vi "Control.vi"(6 "Kp2":dbl, 7 "Q":dbl, 9 "KV":dbl, 10 "Zigmae":dbl[](array[numeric]), 11 "Vr/Wr":dbl[](array[numeric])) -> (2 "W":dbl, 3 "V":dbl)   [LabVIEW 2011]
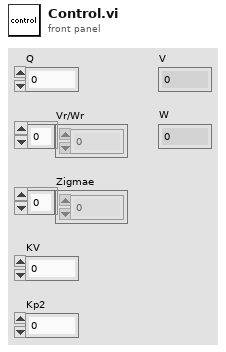
[diagram p1: front panel]
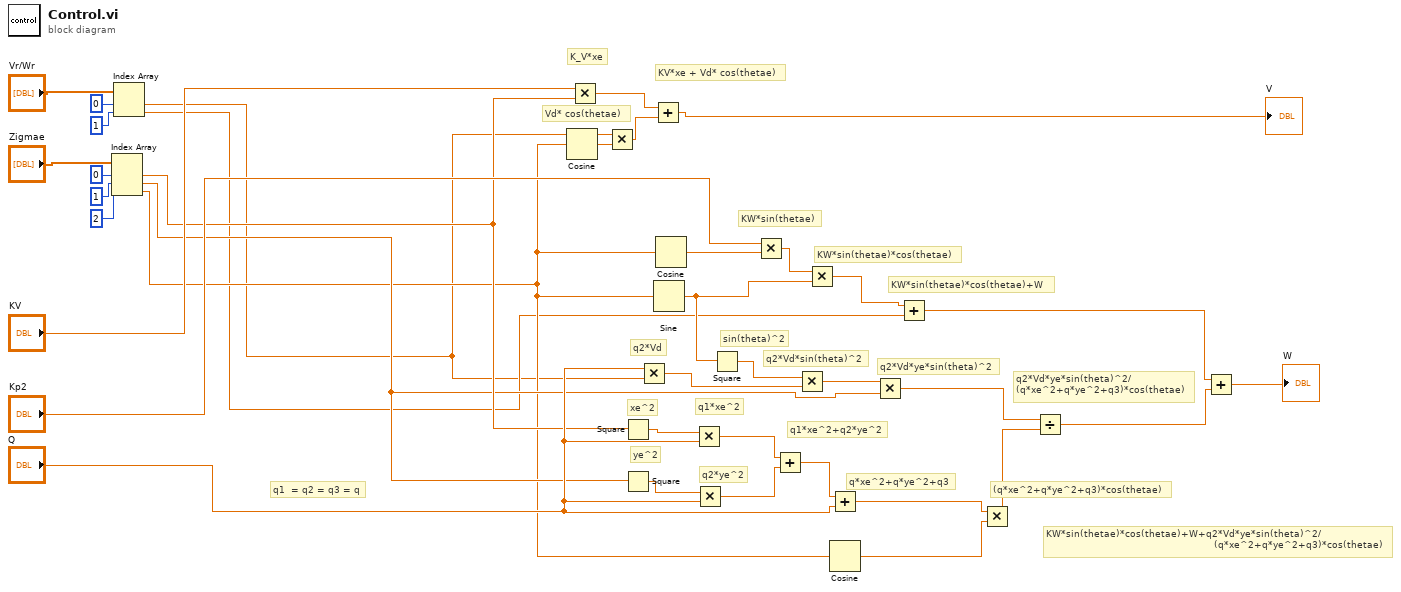
[diagram p0: block diagram]
diagram:
  # "q2*Vd*ye*sin(theta)^2"
  # "KW*sin(thetae)*cos(thetae)+W+q2*Vd*ye*sin(theta)^2/\n                                                        (q*xe^2+q*ye^2+q3)*cos(thetae)"
  # "q2*Vd*ye*sin(theta)^2/\n(q*xe^2+q*ye^2+q3)*cos(thetae)"
  # "(q*xe^2+q*ye^2+q3)*cos(thetae)"
  # "q*xe^2+q*ye^2+q3"
  # "q1*xe^2+q2*ye^2"
  # "q2*ye^2"
  # "q1*xe^2"
  # "ye^2"
  # "xe^2"
  # "q2*Vd*sin(theta)^2"
  # "sin(theta)^2"
  # "q2*Vd"
  # "q1  = q2 = q3 = q"
  # "KW*sin(thetae)*cos(thetae)+W"
  # "KW*sin(thetae)*cos(thetae)"
  # "KW*sin(thetae)"
  # "Vd* cos(thetae)"
  # "KV*xe + Vd* cos(thetae)"
  # "K_V*xe"
  n1 = Index Array(array="Zigmae", index #1=0 ("index"), index #2=1 ("index"), index #3=2 ("index")) -> (element #1=w7:dbl, element #2=w6:dbl, element #3=w5:dbl)
  n2 = Index Array(array="Vr/Wr", index #1=0 ("index"), index #2=1 ("index")) -> (element #1=w3:dbl, element #2=w4:dbl)
  n3 = Cosine(x=w5) -> (cos(x)=w14:dbl)
  n4 = Multiply(x="KV", y=w7) -> (x*y=w13:dbl)
  n5 = Multiply(x=w3, y=w14) -> (x*y=w15:dbl)
  n6 = Square(x=w7) -> (x^2=w22:dbl)
  n7 = Square(x=w6) -> (x^2=w23:dbl)
  n8 = Multiply(x="Q", y=w3) -> (x*y=w21:dbl)
  n9 = Add(x=w13, y=w15) -> (x+y=→"V":dbl)
  n10 = Sine(x=w5) -> (sin(x)=w19:dbl)
  n11 = Cosine(x=w5) -> (cos(x)=w16:dbl)
  n12 = Multiply(x=w22, y="Q") -> (x*y=w25:dbl)
  n13 = Multiply(x=w23, y="Q") -> (x*y=w24:dbl)
  n14 = Square(x=w19) -> (x^2=w20:dbl)
  n15 = Multiply(x="Kp2", y=w16) -> (x*y=w17:dbl)
  n16 = Add(x=w25, y=w24) -> (x+y=w26:dbl)
  n17 = Multiply(x=w20, y=w21) -> (x*y=w12:dbl)
  n18 = Multiply(x=w17, y=w19) -> (x*y=w18:dbl)
  n19 = Add(x=w26, y="Q") -> (x+y=w28:dbl)
  n20 = Cosine(x=w5) -> (cos(x)=w27:dbl)
  n21 = Multiply(x=w12, y=w6) -> (x*y=w11:dbl)
  n22 = Add(x=w18, y=w4) -> (x+y=w31:dbl)
  n23 = Multiply(x=w28, y=w27) -> (x*y=w29:dbl)
  n24 = Divide(x=w11, y=w29) -> (x/y=w30:dbl)
  n25 = Add(x=w31, y=w30) -> (x+y=→"W":dbl)
